vi "switchDevice.vi"(8 "error in (no error)":errorcluster, 9 "on":bool, 10 "use_common_on_off":bool, 11 "Xcite in":refnum<class "Xcite.lvclass">) -> (0 "error out":errorcluster, 3 "Xcite out":refnum<class "Xcite.lvclass">)   [LabVIEW 2019, in "Xcite.lvclass"]
doc: "Master switch for device output"
uses:
  Xcite.lvclass
  Xcite.lvclass/Xcite.ctl
  etc.xcite/XCite.lvlib
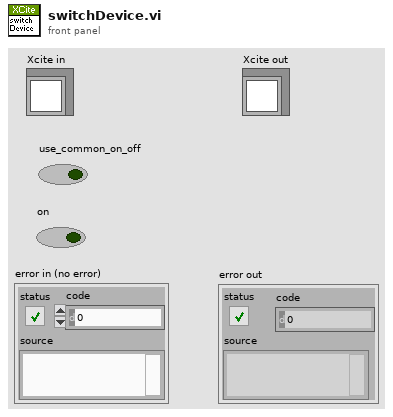
[diagram p1: front panel]
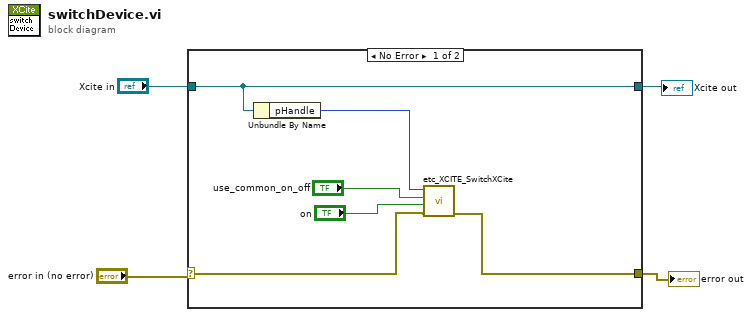
[diagram p0: block diagram]
diagram:
  n1 = case shown="No Error" "error in (no error)" {
    selector: "error in (no error)" -> [w10 w12]
    tunnel: [w9 w12] -> w3
    tunnel: "Xcite in" -> [w6 w11]
    tunnel: [w6 w11] -> w1
    frame No Error {
      n2 = Unbundle By Name(w6) -> ("pHandle"=w5:u64)
      n3 = call "etc_XCITE_SwitchXCite.vi"("error in (no error)"=w10, "bOn"="on", "bUseCommonOnOff"="use_common_on_off", "h"=w5) -> ("error out"=w9:errorcluster)  [unwired: 5 in, 2 out]
    }
    frame Error {
    }
  }
  "Xcite out" <- w1
  "error out" <- w3
